vi "Shutdown.vi"(8 "error in (no error)":errorcluster, 11 "Axsun_1310_SS in":refnum<class "Axsun_1310_SS.lvclass">) -> (0 "error out":errorcluster, 3 "Axsun_1310_SS out":refnum<class "Axsun_1310_SS.lvclass">)   [LabVIEW 2015, in "Axsun_1310_SS.lvclass"]
uses:
  Axsun_1310_SS.lvclass
  Axsun_1310_SS.lvclass/Axsun_1310_SS.ctl
  C:/Program Files (x86)/Axsun/Axsun OCT Control/AxsunOCTControl.dll
  Laser.lvclass
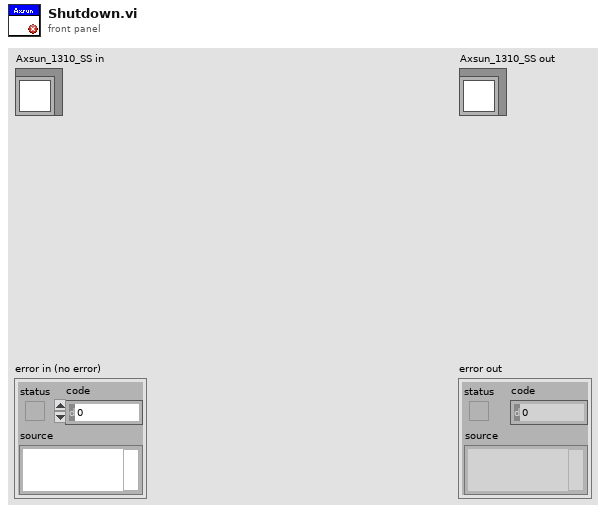
[diagram p1: front panel]
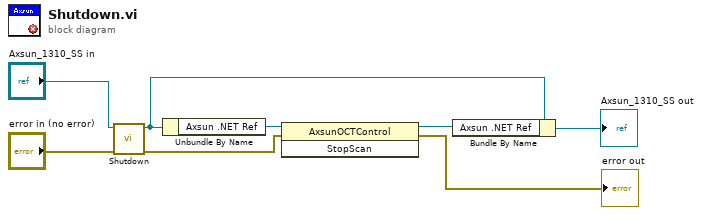
[diagram p0: block diagram]
diagram:
  n1 = call-parent "Shutdown.vi"("error in (no error)"="error in (no error)", "Laser in"="Axsun_1310_SS in") -> ("error out"=w5:errorcluster, "Laser out"=w4:refnum<class "Axsun_1310_SS.lvclass">)  [unwired: 8 in]
  n2 = Unbundle By Name(w4) -> ("Axsun .NET Ref"=w6:refnum<k24>)
  n3 = invoke class="AxsunOCTControl" method="StopScan"(reference=w6, error in=w5) -> (reference out=w3:refnum<k24>, error out=→"error out":errorcluster)  [unwired: 1 in, 1 out]
  n4 = Bundle By Name(cluster=w4, "Axsun .NET Ref"=w3) -> (→"Axsun_1310_SS out":refnum<class "Axsun_1310_SS.lvclass">)
